vi "x-axis.vi"(8 "error in (no error)":errorcluster, 11 "Analog Out Scan in":refnum<class "Analog Out Scan.lvclass">) -> (0 "error out":errorcluster, 1 "Label":string, 2 "Unit":string, 3 "Analog Out Scan out":refnum<class "Analog Out Scan.lvclass">)   [LabVIEW 2009, in "Analog Out Scan.lvclass"]
uses:
  Analog Out Scan.lvclass
  Scanner/Scanner.lvclass
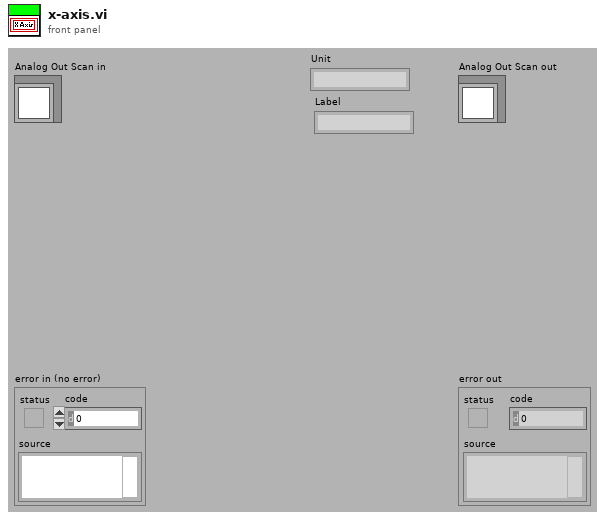
[diagram p1: front panel]
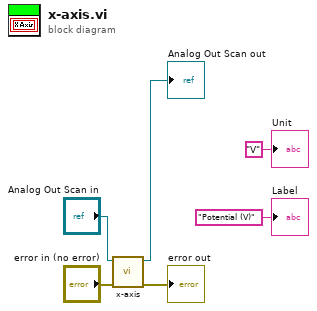
[diagram p0: block diagram]
diagram:
  n1 = call-parent "x-axis.vi"("error in (no error)"="error in (no error)", "Scanner in"="Analog Out Scan in") -> ("error out"=→"error out":errorcluster, "Scanner out"=→"Analog Out Scan out":refnum<class "Analog Out Scan.lvclass">)  [unwired: 6 in, 2 out]
  "Label" <- "Potential (V)" ("Label")
  "Unit" <- "V" ("Unit")
